vi "Stop_get.vi"(8 "error in (no error)":errorcluster) -> (0 "error out":errorcluster, 2 "Stop":bool)   [LabVIEW 2009, in "NetworkVar.lvlib"]
uses:
  NetworkVar.lvlib
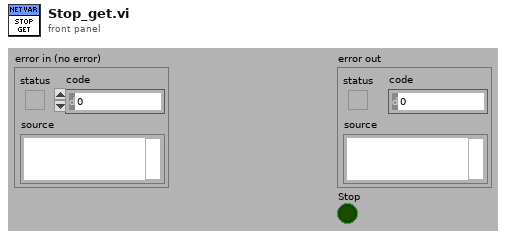
[diagram p1: front panel]
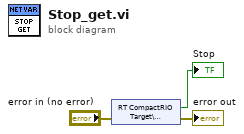
[diagram p0: block diagram]
diagram:
  n1 = shared-variable "RT CompactRIO Target\\NetworkVar.lvlib\\Stop"(error in="error in (no error)") -> (→"Stop":bool, error out=→"error out":errorcluster)
